vi "探头校准标准值显示.vi"(11 "校准参数":u16(ring) caption="校准参数：" items=["pH", "DO", "浊度", "电导率", "叶绿素a", "藻密度", "ORP", "DO2"]) -> (1 "标液三":sgl, 2 "标液二":sgl, 3 "标液一":sgl)   [LabVIEW 2016, in "斯坦道多参数.lvlib"]
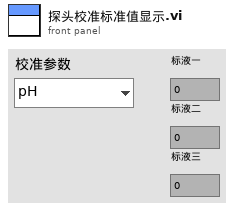
[diagram p1: front panel]
types:
  T1 = typedef "斯坦道多参数.lvlib/探头类型.ctl" = enum16{"禹山", "国弘", "纳清", "STD"}
  T2 = cluster{"pH探头选择":T1, "DO探头选择":T1, "电导率探头选择":T1, "浊度探头选择":T1, "悬浮物探头选择":T1, "叶绿素a探头选择":T1, "蓝绿藻探头选择":T1, "orp探头选择":T1, "COD探头选择":T1, "DO2探头选择":T1, "氨氮探头选择":T1, "水中油探头选择":T1, "余氯探头选择":T1}
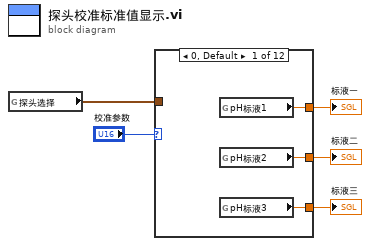
[diagram p0: block diagram]
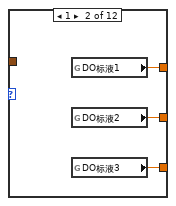
[diagram p2: hidden frame]
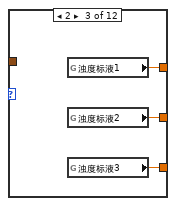
[diagram p3: hidden frame]
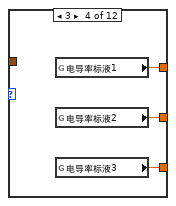
[diagram p4: hidden frame]
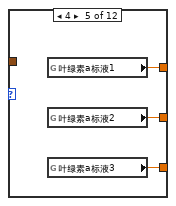
[diagram p5: hidden frame]
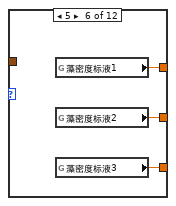
[diagram p6: hidden frame]
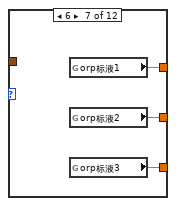
[diagram p7: hidden frame]
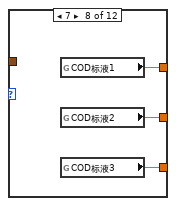
[diagram p8: hidden frame]
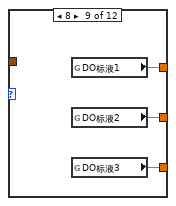
[diagram p9: hidden frame]
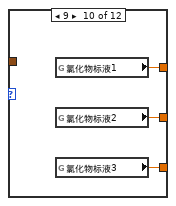
[diagram p10: hidden frame]
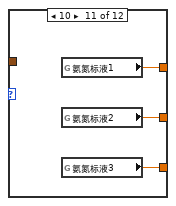
[diagram p11: hidden frame]
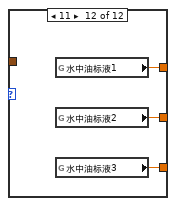
[diagram p12: hidden frame]
diagram:
  n1 = global read "断电保存变量.vi" "探头选择"() -> (w3:T2)
  n2 = case shown="0, Default" "校准参数" {
    tunnel: [w8 w11 w14 w17 w18 w22 w24 w29 w32 w35 w38 w41] -> w5
    tunnel: w3 -> [_ _ _ _ _ _ _ _ _ _ _ _]
    tunnel: [w7 w10 w13 w16 w19 w21 w25 w28 w31 w34 w37 w40] -> w2
    tunnel: [w6 w9 w12 w15 w20 w23 w26 w27 w30 w33 w36 w39] -> w1
    frame 0, Default {
      n3 = global read "断电保存变量.vi" "pH标液1"() -> (w8:dbl)
      n4 = global read "断电保存变量.vi" "pH标液2"() -> (w7:dbl)
      n5 = global read "断电保存变量.vi" "pH标液3"() -> (w6:dbl)
    }
    frame 1 {
      n6 = global read "断电保存变量.vi" "DO标液1"() -> (w11:dbl)
      n7 = global read "断电保存变量.vi" "DO标液2"() -> (w10:dbl)
      n8 = global read "断电保存变量.vi" "DO标液3"() -> (w9:dbl)
    }
    frame 2 {
      n9 = global read "断电保存变量.vi" "浊度标液1"() -> (w14:dbl)
      n10 = global read "断电保存变量.vi" "浊度标液2"() -> (w13:dbl)
      n11 = global read "断电保存变量.vi" "浊度标液3"() -> (w12:dbl)
    }
    frame 3 {
      n12 = global read "断电保存变量.vi" "电导率标液1"() -> (w17:dbl)
      n13 = global read "断电保存变量.vi" "电导率标液2"() -> (w16:dbl)
      n14 = global read "断电保存变量.vi" "电导率标液3"() -> (w15:dbl)
    }
    frame 4 {
      n15 = global read "断电保存变量.vi" "叶绿素a标液1"() -> (w18:dbl)
      n16 = global read "断电保存变量.vi" "叶绿素a标液2"() -> (w19:dbl)
      n17 = global read "断电保存变量.vi" "叶绿素a标液3"() -> (w20:dbl)
    }
    frame 5 {
      n18 = global read "断电保存变量.vi" "藻密度标液1"() -> (w22:dbl)
      n19 = global read "断电保存变量.vi" "藻密度标液2"() -> (w21:dbl)
      n20 = global read "断电保存变量.vi" "藻密度标液3"() -> (w23:dbl)
    }
    frame 6 {
      n21 = global read "断电保存变量.vi" "orp标液1"() -> (w24:dbl)
      n22 = global read "断电保存变量.vi" "orp标液2"() -> (w25:dbl)
      n23 = global read "断电保存变量.vi" "orp标液3"() -> (w26:dbl)
    }
    frame 7 {
      n24 = global read "断电保存变量.vi" "COD标液1"() -> (w29:dbl)
      n25 = global read "断电保存变量.vi" "COD标液2"() -> (w28:dbl)
      n26 = global read "断电保存变量.vi" "COD标液3"() -> (w27:dbl)
    }
    frame 8 {
      n27 = global read "断电保存变量.vi" "DO标液1"() -> (w32:dbl)
      n28 = global read "断电保存变量.vi" "DO标液2"() -> (w31:dbl)
      n29 = global read "断电保存变量.vi" "DO标液3"() -> (w30:dbl)
    }
    frame 9 {
      n30 = global read "断电保存变量.vi" "氯化物标液1"() -> (w35:dbl)
      n31 = global read "断电保存变量.vi" "氯化物标液2"() -> (w34:dbl)
      n32 = global read "断电保存变量.vi" "氯化物标液3"() -> (w33:dbl)
    }
    frame 10 {
      n33 = global read "断电保存变量.vi" "氨氮标液1"() -> (w38:dbl)
      n34 = global read "断电保存变量.vi" "氨氮标液2"() -> (w37:dbl)
      n35 = global read "断电保存变量.vi" "氨氮标液3"() -> (w36:dbl)
    }
    frame 11 {
      n36 = global read "断电保存变量.vi" "水中油标液1"() -> (w41:dbl)
      n37 = global read "断电保存变量.vi" "水中油标液2"() -> (w40:dbl)
      n38 = global read "断电保存变量.vi" "水中油标液3"() -> (w39:dbl)
    }
  }
  "标液一" <- w5
  "标液二" <- w2
  "标液三" <- w1
